vi "append_to_file.vi"(1 "error in (no error)":errorcluster, 2 "text":string, 3 "file_path":path) -> (0 "error out":errorcluster)   [LabVIEW 2018]
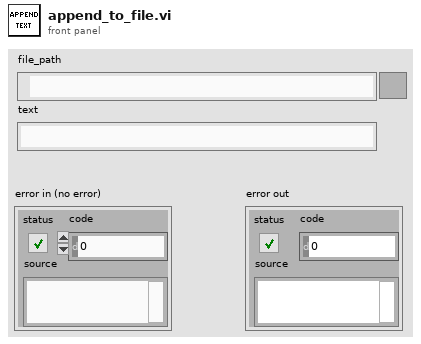
[diagram p1: front panel]
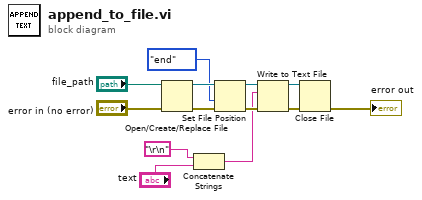
[diagram p0: block diagram]
diagram:
  n1 = Open/Create/Replace File(file path (use dialog)="file_path", error in="error in (no error)") -> (refnum out=w12:refnum<file>, error out=w9:errorcluster)  [unwired: 4 in, 1 out]
  n2 = Concatenate Strings("\r\n", "text") -> (w5:string)
  n3 = Set File Position(refnum=w12, from (0:start)=enum16{"start", "end", "current"}."end", error in=w9) -> (refnum out=w11:refnum<file>, error out=w8:errorcluster)  [unwired: 1 in]
  n4 = Write to Text File(file (use dialog)=w11, text=w5, error in=w8) -> (refnum out=w10:refnum<file>, error out=w7:errorcluster)  [unwired: 1 in, 1 out]
  n5 = Close File(refnum=w10, error in=w7) -> (error out=→"error out":errorcluster)  [unwired: 1 out]
